vi "Test Initiate.vi"(0 "Template Tx Test in":refnum<class "niDTS GNSS RF Test.lvclass">, 11 "error in (no error)":errorcluster) -> (4 "Template Tx Test out":refnum<class "niDTS GNSS RF Test.lvclass">, 15 "error out":errorcluster)   [LabVIEW 2015, in "niDTS GNSS.lvlib" / "niDTS GNSS RF Test.lvclass"]
uses:
  niDTS GNSS RF Test.lvclass
  Dut/Includes/niDTS GNSS Dut INC Handle.ctl
  Dut/Objects/BASE_class/niDTS GNSS Dut.lvclass
  Framework/Dut/Objects/BASE_class/niDTS Dut.lvclass
  RiviInstDriver/InstDriver/Objects/InstDriver.lvclass
  RiviInstDriver/niRfsgGprf/Objects/niRfsgGprf.lvclass
  niDTS GNSS.lvlib
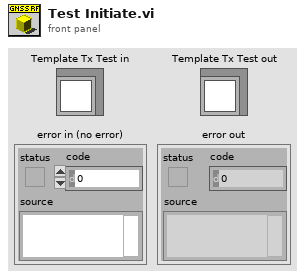
[diagram p1: front panel]
types:
  T1 = typedef "niDTS GNSS.lvlib/niDTS GNSS Dut INC Handle.ctl" = refnum<data-value>
  T2 = typedef "niDTS Framework.lvlib/niDTS Dut INC Handle.ctl" = refnum<data-value>
  T3 = typedef "InstDriver.lvclass/niInstDriver INC Handle.ctl" = refnum<data-value>
  T4 = typedef "niRfsgGprf.lvclass/niRfsgGprf INC Handle.ctl" = refnum<data-value>
  T5 = typedef "niDTS GNSS.lvlib/niDTS GNSS RF Test INC Results.ctl" = cluster{"Measured Frequency (Hz)":dbl, "Mean Frequency Error (Hz)":dbl, "Mean Signal Phase (Deg)":dbl, "Mean Signal Power (dBm)":dbl, "Peak to Average Power Ratio":dbl, "C/No (dB)":dbl, "Max. Power (dBm)":dbl, "Min. Power (dBm)":dbl, "Power Trace":cluster{"Xo":dbl, "dx":dbl, "TxpPowerTrace":string[]}, "IQ Trace":cluster{"Xo":dbl, "dx":dbl, "TxpIQTrace":string[]}, "Phase Trace":cluster{"Xo":dbl, "dx":dbl, "TxpPhaseTrace":string[]}}
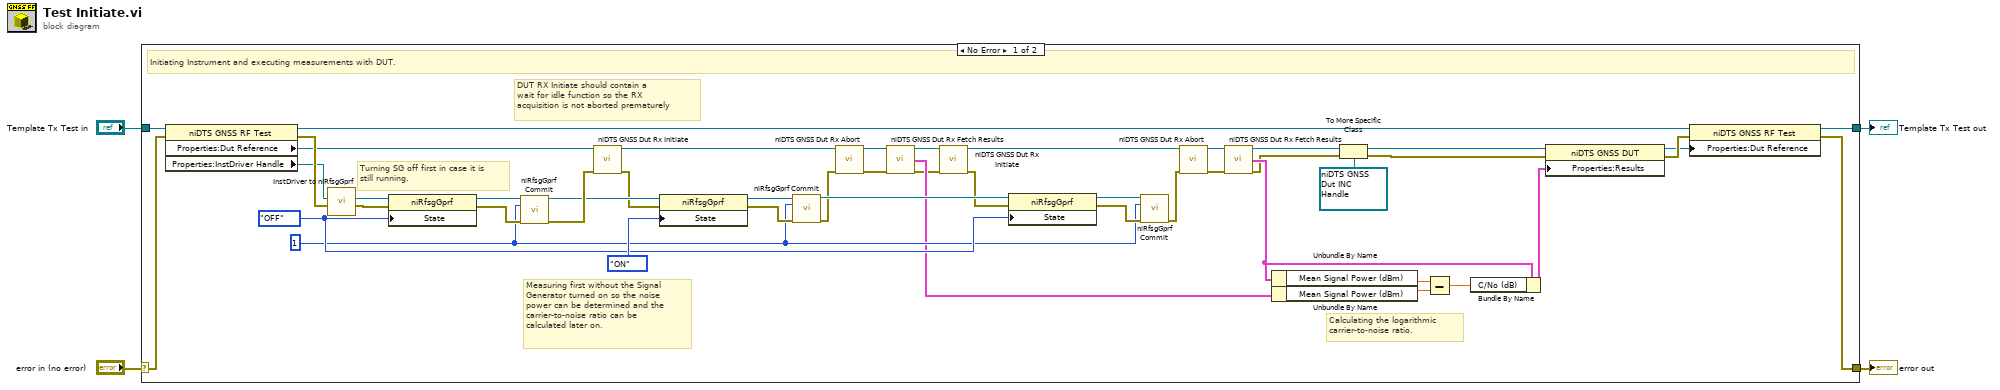
[diagram p0: block diagram]
diagram:
  n1 = case shown="No Error" "error in (no error)" {
    selector: "error in (no error)" -> [w50 w53]
    tunnel: [w12 w53] -> w3
    tunnel: [w13 w52] -> w1
    tunnel: "Template Tx Test in" -> [w51 w52]
    frame No Error {
      w40 = enum16{"OFF", "PENDING", "ON"}."OFF" ("SOURce:RFSG:GPRF:State")
      w39 = 1 ("Driver Instance")
      # "Calculating the logarithmic \ncarrier-to-noise ratio."
      # "Measuring first without the Signal \nGenerator turned on so the noise \npower can be determined and the \ncarrier-to-noise ratio can be \ncalculated later on."
      # "Turning SG off first in case it is \nstill running."
      # "DUT RX Initiate should contain a\nwait for idle function so the RX \nacquisition is not aborted prematurely"
      # "Initiating Instrument and executing measurements with DUT."
      n2 = property class="niDTS GNSS RF Test"(reference=w51, error in=w50) -> (reference out=w15:refnum<class "niDTS GNSS RF Test.lvclass">, error out=w38:errorcluster, "Properties:Dut Reference"=w32:T2, "Properties:InstDriver Handle"=w37:T3)
      n3 = call "InstDriver to niRfsgGprf.vi"("error in (no error)"=w38, "InstDriver Handle in"=w37) -> ("error out"=w35:errorcluster, "InstDriver Handle out"=w36:refnum<data-value>)  [unwired: 8 in]
      n4 = property class="niRfsgGprf"(reference=w36, error in=w35, "State"=w40) -> (reference out=w48:refnum<data-value>, error out=w49:errorcluster)
      n5 = call "niRfsgGprf Commit.vi"("InstDriver Handle in"=w48, "Instance"=w39, "error in (no error)"=w49) -> ("InstDriver Handle out"=w11:T4, "error out"=w34:errorcluster)  [unwired: 11 in]
      n6 = call "niDTS GNSS Dut Rx Initiate.vi"("Dut Handle in"=w32, "error in (no error)"=w34) -> ("Dut Handle out"=w33:T2, "error out"=w10:errorcluster)  [unwired: 12 in]
      n7 = property class="niRfsgGprf"(reference=w11, error in=w10, "State"=enum16{"OFF", "PENDING", "ON"}."ON" ("SOURce:RFSG:GPRF:State")) -> (reference out=w46:T4, error out=w45:errorcluster)
      n8 = call "niRfsgGprf Commit.vi"("InstDriver Handle in"=w46, "Instance"=w39, "error in (no error)"=w45) -> ("InstDriver Handle out"=w41:T4, "error out"=w9:errorcluster)  [unwired: 11 in]
      n9 = call "niDTS GNSS Dut Rx Abort.vi"("Dut Handle in"=w33, "error in (no error)"=w9) -> ("Dut Handle out"=w31:T2, "error out"=w29:errorcluster)  [unwired: 12 in]
      n10 = call "niDTS GNSS Dut Rx Fetch Results.vi"("Dut Handle in"=w31, "error in (no error)"=w29) -> ("Dut Handle out"=w30:T2, "Results"=w26:T5, "error out"=w8:errorcluster)  [unwired: 11 in]
      n11 = call "niDTS GNSS Dut Rx Initiate.vi"("Dut Handle in"=w30, "error in (no error)"=w8) -> ("Dut Handle out"=w44:T2, "error out"=w7:errorcluster)  [unwired: 12 in]
      n12 = property class="niRfsgGprf"(reference=w41, error in=w7, "State"=w40) -> (reference out=w43:T4, error out=w42:errorcluster)
      n13 = call "niRfsgGprf Commit.vi"("InstDriver Handle in"=w43, "Instance"=w39, "error in (no error)"=w42) -> ("error out"=w6:errorcluster)  [unwired: 11 in, 1 out]
      n14 = call "niDTS GNSS Dut Rx Abort.vi"("Dut Handle in"=w44, "error in (no error)"=w6) -> ("Dut Handle out"=w28:T2, "error out"=w27:errorcluster)  [unwired: 12 in]
      n15 = call "niDTS GNSS Dut Rx Fetch Results.vi"("Dut Handle in"=w28, "error in (no error)"=w27) -> ("Dut Handle out"=w21:T2, "Results"=w23:T5, "error out"=w5:errorcluster)  [unwired: 11 in]
      n16 = Unbundle By Name(w23) -> ("Mean Signal Power (dBm)"=w25:dbl)
      n17 = Unbundle By Name(w26) -> ("Mean Signal Power (dBm)"=w24:dbl)
      n18 = To More Specific Class(target class=T1 refnum ("GNSS Dut Handle"), reference=w21, error in=w5) -> (specific class reference=w19:T1, error out=w18:errorcluster)
      n19 = Subtract(x=w25, y=w24) -> (x-y=w22:dbl)
      n20 = Bundle By Name(cluster=w23, "C/No (dB)"=w22) -> (w17:T5)
      n21 = property class="niDTS GNSS DUT"(reference=w19, error in=w18, "Properties:Results"=w17) -> (reference out=w14:T1, error out=w16:errorcluster)
      n22 = property class="niDTS GNSS RF Test"(reference=w15, error in=w16, "Properties:Dut Reference"=w14) -> (reference out=w13:refnum<class "niDTS GNSS RF Test.lvclass">, error out=w12:errorcluster)
    }
    frame Error {
    }
  }
  "error out" <- w3
  "Template Tx Test out" <- w1
